vi "Control File.vi"(4 "Description":string, 6 "Display Name":string, 7 "Maintainer":string, 8 "error in (no error)":errorcluster, 9 "Version":string, 10 "Package Name":string, 11 "Stage Path":path) -> (0 "error out":errorcluster, 3 "Stage Path Out":path)   [LabVIEW 2016]
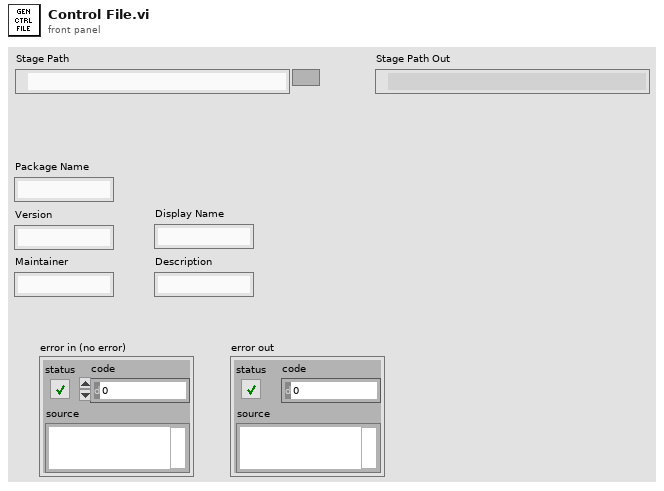
[diagram p1: front panel]
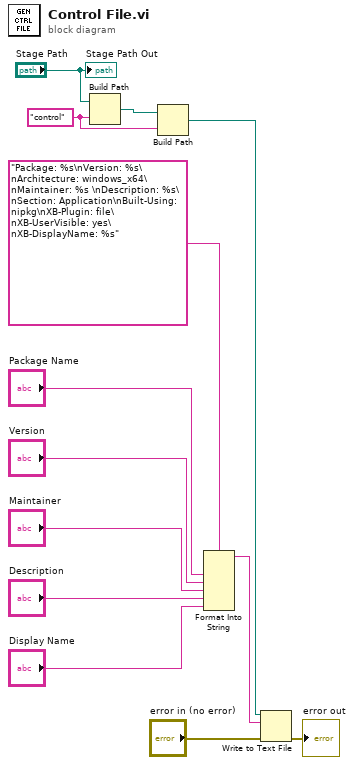
[diagram p0: block diagram]
diagram:
  w4 = "control" ("name or relative path")
  n1 = Build Path(base path="Stage Path", name or relative path=w4) -> (appended path=w5:path)
  n2 = Build Path(base path=w5, name or relative path=w4) -> (appended path=w3:path)
  n3 = Format Into String(format string="Package: %s\nVersion: %s\nArchitecture: windows_x64\nMaintainer: %s \nDescription: %s\nSection: Application\nBuilt-Using: nipkg\nXB-Plugin: file\nXB-UserVisible: yes\nXB-DisplayName: %s", "Package Name", "Version", "Maintainer", "Description", "Display Name") -> (resulting string=w6:string)  [unwired: 2 in, 1 out]
  n4 = Write to Text File(file (use dialog)=w3, text=w6, error in="error in (no error)") -> (error out=→"error out":errorcluster)  [unwired: 1 in, 2 out]
  "Stage Path Out" <- "Stage Path"
